vi "Program31.vi"() -> ()   [LabVIEW 2020]
panel:
  in  "stop":bool
  in  "Color Box 2":u32(colorbox)
  in  "Plot Area:Colors:BG Color":u32(colorbox)
  out "Waveform Graph":dbl[][](graph)
  in  "Plot.Point Style":u8
  in  "X Scale.Name Label.Text":string
  in  "Plot.Plot Name 2":string
  in  "Plot.Plot Name":string
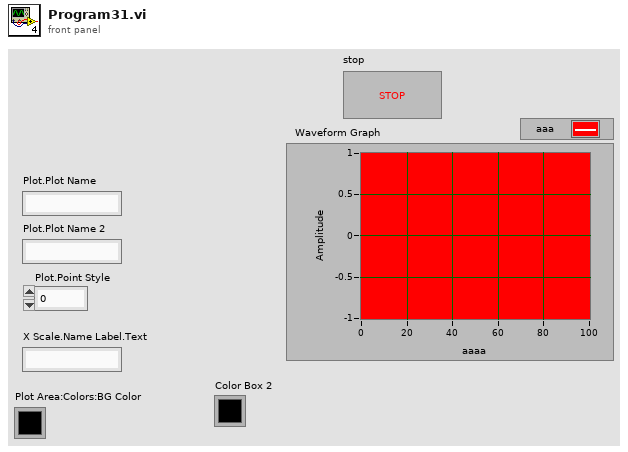
[diagram p1: front panel]
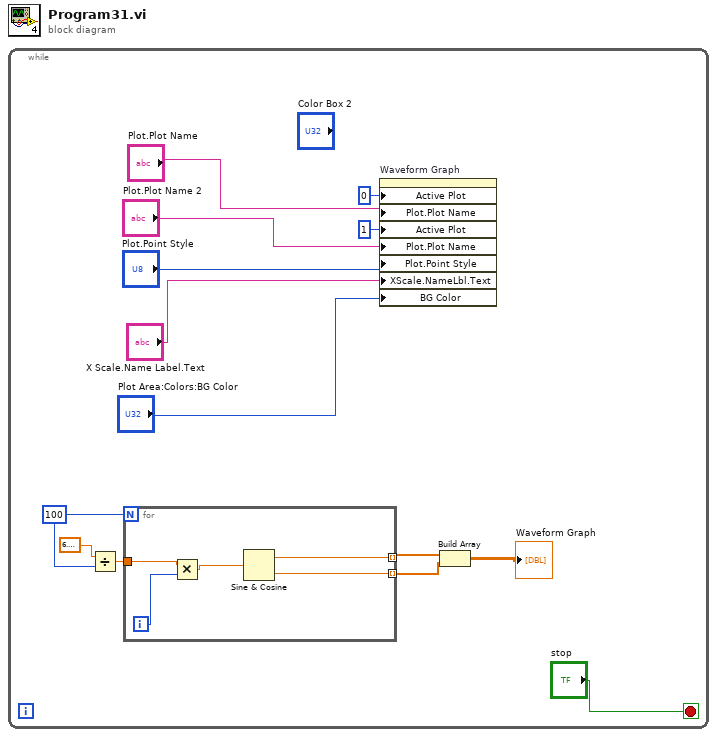
[diagram p0: block diagram]
diagram:
  n1 = while {
    stop <- "stop" stop-if-true
    w7 = 100
    n2 = Divide(x=6.283185307179586, y=w7) -> (x/y=w5:dbl)
    n3 = for {
      N: w7 -> [_]
      tunnel: w5 -> [w19]
      tunnel: [w16] -> w3 mode=indexing
      tunnel: [w15] -> w4 mode=indexing
      i -> [w18]
      n4 = Multiply(x=w19, y=w18) -> (x*y=w17:dbl)
      n5 = Sine & Cosine(0:w17) -> (1:w16:dbl, 2:w15:dbl)
    }
    n6 = property on="Waveform Graph" class="WFGraph (strict)"("Active Plot"=u32 0, "Plot.Plot Name"="Plot.Plot Name", "Active Plot"=u32 1, "Plot.Plot Name"="Plot.Plot Name 2", "Plot.Point Style"="Plot.Point Style", "XScale.NameLbl.Text"="X Scale.Name Label.Text", "BG Color"="Plot Area:Colors:BG Color") -> ()  [unwired: 2 in, 2 out]
    n7 = Build Array(w3, w4) -> (→"Waveform Graph":dbl[][])
  }
